vi "メイン.vi"() -> (2 "測定周期/ms":dbl, 3 "値転記用配列":T2[](array[typedef]))   [LabVIEW 2021] (continued)
                frame 8 {
                  n4757 = local write "測定新値\nリセット用 9"(w7303) -> ()
                  n4758 = local write "測定旧値 9"(w7303) -> ()
                }
                frame 9 {
                  n4759 = local write "測定新値\nリセット用 10"(w7304) -> ()
                  n4760 = local write "測定旧値 10"(w7304) -> ()
                }
                frame 10 {
                  n4761 = local write "測定新値\nリセット用 11"(w7305) -> ()
                  n4762 = local write "測定旧値 11"(w7305) -> ()
                }
                frame 11 {
                  n4763 = local write "測定新値\nリセット用 12"(w7306) -> ()
                  n4764 = local write "測定旧値 12"(w7306) -> ()
                }
              }
            }
          }
          frame #2 {
            # "⑤キュー"
            # "④グローバル_測定キャンセルボタンを\n対象測定新値がFalseならTrueにする"
            n4765 = case shown="TRUE" w7309 {
              tunnel: [_ w7319] -> w7313
              tunnel: w7312 -> [_ w7318]
              tunnel: [_ w7317] -> w7311
              tunnel: w7310 -> [_ w7316]
              tunnel: [w7314 w7315] -> w7308
              tunnel: [w7314 w7315] -> w7307
              frame False {
                w7314 = TRUE
              }
              frame True {
                w7315 = TRUE
                n4766 = Enqueue Element(queue=w7318, element="測定1", error in (no error)=w7316) -> (queue out=w7319:refnum<queue>, error out=w7317:errorcluster)  [unwired: 1 in, 1 out]
              }
            }
            n4767 = local write "G_メイン測定キャンセルボタン"(w7308) -> ()
            n4768 = global write "測定キャンセルボタン.vi" "グローバル_測定キャンセルボタン"(w7307) -> ()
          }
        }
        n4769 = for {
          N: 12 -> [_]
          tunnel: w7211 -> [w7225]
          i -> [w7226]
          n4770 = case shown="0, デフォルト" w7226 {
            tunnel: w7225 -> [w7227 w7228 w7229 w7230 w7231 w7232 w7233 w7234 w7235 w7236 w7237 w7238]
            frame 0, Default {
              n4771 = property on="メイン測定ボタン_単発 1" class="Bool (指定)"("DisabledEnum"=w7227) -> ()  [unwired: 2 in, 2 out]
              n4772 = property on="メイン測定ボタン_連続 1" class="Bool (指定)"("DisabledEnum"=w7227) -> ()  [unwired: 2 in, 2 out]
            }
            frame 1 {
              n4773 = property on="メイン測定ボタン_単発 2" class="Bool (指定)"("DisabledEnum"=w7228) -> ()  [unwired: 2 in, 2 out]
              n4774 = property on="メイン測定ボタン_連続 2" class="Bool (指定)"("DisabledEnum"=w7228) -> ()  [unwired: 2 in, 2 out]
            }
            frame 2 {
              n4775 = property on="メイン測定ボタン_単発 3" class="Bool (指定)"("DisabledEnum"=w7229) -> ()  [unwired: 2 in, 2 out]
              n4776 = property on="メイン測定ボタン_連続 3" class="Bool (指定)"("DisabledEnum"=w7229) -> ()  [unwired: 2 in, 2 out]
            }
            frame 3 {
              n4777 = property on="メイン測定ボタン_単発 4" class="Bool (指定)"("DisabledEnum"=w7230) -> ()  [unwired: 2 in, 2 out]
              n4778 = property on="メイン測定ボタン_連続 4" class="Bool (指定)"("DisabledEnum"=w7230) -> ()  [unwired: 2 in, 2 out]
            }
            frame 4 {
              n4779 = property on="メイン測定ボタン_単発 5" class="Bool (指定)"("DisabledEnum"=w7231) -> ()  [unwired: 2 in, 2 out]
              n4780 = property on="メイン測定ボタン_連続 5" class="Bool (指定)"("DisabledEnum"=w7231) -> ()  [unwired: 2 in, 2 out]
            }
            frame 5 {
              n4781 = property on="メイン測定ボタン_連続 6" class="Bool (指定)"("DisabledEnum"=w7232) -> ()  [unwired: 2 in, 2 out]
              n4782 = property on="メイン測定ボタン_単発 6" class="Bool (指定)"("DisabledEnum"=w7232) -> ()  [unwired: 2 in, 2 out]
            }
            frame 6 {
              n4783 = property on="メイン測定ボタン_連続 7" class="Bool (指定)"("DisabledEnum"=w7233) -> ()  [unwired: 2 in, 2 out]
              n4784 = property on="メイン測定ボタン_単発 7" class="Bool (指定)"("DisabledEnum"=w7233) -> ()  [unwired: 2 in, 2 out]
            }
            frame 7 {
              n4785 = property on="メイン測定ボタン_単発 8" class="Bool (指定)"("DisabledEnum"=w7234) -> ()  [unwired: 2 in, 2 out]
              n4786 = property on="メイン測定ボタン_連続 8" class="Bool (指定)"("DisabledEnum"=w7234) -> ()  [unwired: 2 in, 2 out]
            }
            frame 8 {
              n4787 = property on="メイン測定ボタン_単発 9" class="Bool (指定)"("DisabledEnum"=w7235) -> ()  [unwired: 2 in, 2 out]
              n4788 = property on="メイン測定ボタン_連続 9" class="Bool (指定)"("DisabledEnum"=w7235) -> ()  [unwired: 2 in, 2 out]
            }
            frame 9 {
              n4789 = property on="メイン測定ボタン_単発 10" class="Bool (指定)"("DisabledEnum"=w7236) -> ()  [unwired: 2 in, 2 out]
              n4790 = property on="メイン測定ボタン_連続 10" class="Bool (指定)"("DisabledEnum"=w7236) -> ()  [unwired: 2 in, 2 out]
            }
            frame 10 {
              n4791 = property on="メイン測定ボタン_単発 11" class="Bool (指定)"("DisabledEnum"=w7237) -> ()  [unwired: 2 in, 2 out]
              n4792 = property on="メイン測定ボタン_連続 11" class="Bool (指定)"("DisabledEnum"=w7237) -> ()  [unwired: 2 in, 2 out]
            }
            frame 11 {
              n4793 = property on="メイン測定ボタン_連続 12" class="Bool (指定)"("DisabledEnum"=w7238) -> ()  [unwired: 2 in, 2 out]
              n4794 = property on="メイン測定ボタン_単発 12" class="Bool (指定)"("DisabledEnum"=w7238) -> ()  [unwired: 2 in, 2 out]
            }
          }
        }
        n4795 = property on="TOPページへ" class="Bool"("DisabledEnum"=w7211) -> ()  [unwired: 2 in, 2 out]
        n4796 = property on="保存して終了" class="Bool"("DisabledEnum"=w7211) -> ()  [unwired: 2 in, 2 out]
        n4797 = property on="保存せずに" class="Bool"("DisabledEnum"=w7211) -> ()  [unwired: 2 in, 2 out]
      }
      event Value Change {
        w7322 = T8."Disabled" ("無効")
        # "※複製時\n①このボタンで操作する以外の\n測定旧値\n測定新値\nを複製して作る\n②ある分だけの\nを複製して作る\n③複製した番号未満のケースに\n②をコピーして置き換える\n(編集より楽な為)\n④はそのまま\n⑤測定新値の\nボタンが複製されているか確認\n⑥Ⅰ.初期設定の\n測定新値_リセットの初期化\nを必ず作る事\n⑦キュー"
        # "⑤"
        n4798 = event-data() -> ("NewVal"=w7331:T7)  [unwired: 1 in, 2 out]
        "測定新値 2" <- w7331
        n4799 = local read "書込周期/ms"() -> (w7321:dbl)
        n4800 = Wait (ms)(milliseconds to wait=w7321) -> ()  [unwired: 1 out]
        n4801 = flat-sequence {
          tunnel: [w7353] -> w7327
          tunnel: [w7352] -> w7326
          tunnel: [w7351] -> w7325
          tunnel: [w7350] -> w7324
          tunnel: w7331 -> [w7351]
          tunnel: w7332 -> [w7352]
          tunnel: w7334 -> [w7353]
          tunnel: [w7403] -> w7330
          tunnel: [w7402] -> w7329
          tunnel: [w7401] -> w7328
          tunnel: w7327 -> [w7403]
          tunnel: w7326 -> [w7402]
          tunnel: w7325 -> [w7401]
          tunnel: w7324 -> [w7399]
          tunnel: [w7424] -> w7335
          tunnel: [w7422] -> w7333
          tunnel: w7330 -> [w7423]
          tunnel: w7329 -> [w7421]
          tunnel: w7328 -> [w7420]
          frame #0 {
            w7350 = 32
            # "測定旧値・新値～32までTrueだったらMAX/MINグローバルリセット"
            # "①"
            n4802 = for {
              N: w7350 -> [_]
              i -> [w7354]
              n4803 = case shown="11" w7354 {
                frame 0, Default {
                  n4804 = local read "測定新値\nリセット用 1"() -> (w7355:bool)
                  n4805 = local read "測定旧値 1"() -> (w7356:bool)
                  n4806 = case shown="FALSE" w7355 {
                    frame False {
                    }
                    frame True {
                      n4807 = property on="MAX/MINグローバルリセット用" class="Arr (指定)"() -> ("Value"=w7357:string[][])  [unwired: 2 in, 2 out]
                      n4808 = global write "測定値MAXMIN_G.vi" "測定値MAX/MINグローバル"(w7357) -> ()
                    }
                  }
                  n4809 = case shown="FALSE" w7356 {
                    frame False {
                    }
                    frame True {
                      n4810 = property on="MAX/MINグローバルリセット用" class="Arr (指定)"() -> ("Value"=w7358:string[][])  [unwired: 2 in, 2 out]
                      n4811 = global write "測定値MAXMIN_G.vi" "測定値MAX/MINグローバル"(w7358) -> ()
                    }
                  }
                }
                frame 2 {
                  n4812 = local read "測定新値\nリセット用 3"() -> (w7359:bool)
                  n4813 = local read "測定旧値 3"() -> (w7360:bool)
                  n4814 = case shown="FALSE" w7359 {
                    frame False {
                    }
                    frame True {
                      n4815 = property on="MAX/MINグローバルリセット用" class="Arr (指定)"() -> ("Value"=w7361:string[][])  [unwired: 2 in, 2 out]
                      n4816 = global write "測定値MAXMIN_G.vi" "測定値MAX/MINグローバル"(w7361) -> ()
                    }
                  }
                  n4817 = case shown="FALSE" w7360 {
                    frame False {
                    }
                    frame True {
                      n4818 = property on="MAX/MINグローバルリセット用" class="Arr (指定)"() -> ("Value"=w7362:string[][])  [unwired: 2 in, 2 out]
                      n4819 = global write "測定値MAXMIN_G.vi" "測定値MAX/MINグローバル"(w7362) -> ()
                    }
                  }
                }
                frame 3 {
                  n4820 = local read "測定新値\nリセット用 4"() -> (w7363:bool)
                  n4821 = local read "測定旧値 4"() -> (w7364:bool)
                  n4822 = case shown="FALSE" w7363 {
                    frame False {
                    }
                    frame True {
                      n4823 = property on="MAX/MINグローバルリセット用" class="Arr (指定)"() -> ("Value"=w7365:string[][])  [unwired: 2 in, 2 out]
                      n4824 = global write "測定値MAXMIN_G.vi" "測定値MAX/MINグローバル"(w7365) -> ()
                    }
                  }
                  n4825 = case shown="FALSE" w7364 {
                    frame False {
                    }
                    frame True {
                      n4826 = property on="MAX/MINグローバルリセット用" class="Arr (指定)"() -> ("Value"=w7366:string[][])  [unwired: 2 in, 2 out]
                      n4827 = global write "測定値MAXMIN_G.vi" "測定値MAX/MINグローバル"(w7366) -> ()
                    }
                  }
                }
                frame 4 {
                  n4828 = local read "測定新値\nリセット用 5"() -> (w7367:bool)
                  n4829 = local read "測定旧値 5"() -> (w7368:bool)
                  n4830 = case shown="FALSE" w7367 {
                    frame False {
                    }
                    frame True {
                      n4831 = property on="MAX/MINグローバルリセット用" class="Arr (指定)"() -> ("Value"=w7369:string[][])  [unwired: 2 in, 2 out]
                      n4832 = global write "測定値MAXMIN_G.vi" "測定値MAX/MINグローバル"(w7369) -> ()
                    }
                  }
                  n4833 = case shown="FALSE" w7368 {
                    frame False {
                    }
                    frame True {
                      n4834 = property on="MAX/MINグローバルリセット用" class="Arr (指定)"() -> ("Value"=w7370:string[][])  [unwired: 2 in, 2 out]
                      n4835 = global write "測定値MAXMIN_G.vi" "測定値MAX/MINグローバル"(w7370) -> ()
                    }
                  }
                }
                frame 5 {
                  n4836 = local read "測定新値\nリセット用 6"() -> (w7371:bool)
                  n4837 = local read "測定旧値 6"() -> (w7372:bool)
                  n4838 = case shown="FALSE" w7371 {
                    frame False {
                    }
                    frame True {
                      n4839 = property on="MAX/MINグローバルリセット用" class="Arr (指定)"() -> ("Value"=w7373:string[][])  [unwired: 2 in, 2 out]
                      n4840 = global write "測定値MAXMIN_G.vi" "測定値MAX/MINグローバル"(w7373) -> ()
                    }
                  }
                  n4841 = case shown="FALSE" w7372 {
                    frame False {
                    }
                    frame True {
                      n4842 = property on="MAX/MINグローバルリセット用" class="Arr (指定)"() -> ("Value"=w7374:string[][])  [unwired: 2 in, 2 out]
                      n4843 = global write "測定値MAXMIN_G.vi" "測定値MAX/MINグローバル"(w7374) -> ()
                    }
                  }
                }
                frame 6 {
                  n4844 = local read "測定新値\nリセット用 7"() -> (w7375:bool)
                  n4845 = local read "測定旧値 7"() -> (w7376:bool)
                  n4846 = case shown="FALSE" w7375 {
                    frame False {
                    }
                    frame True {
                      n4847 = property on="MAX/MINグローバルリセット用" class="Arr (指定)"() -> ("Value"=w7377:string[][])  [unwired: 2 in, 2 out]
                      n4848 = global write "測定値MAXMIN_G.vi" "測定値MAX/MINグローバル"(w7377) -> ()
                    }
                  }
                  n4849 = case shown="FALSE" w7376 {
                    frame False {
                    }
                    frame True {
                      n4850 = property on="MAX/MINグローバルリセット用" class="Arr (指定)"() -> ("Value"=w7378:string[][])  [unwired: 2 in, 2 out]
                      n4851 = global write "測定値MAXMIN_G.vi" "測定値MAX/MINグローバル"(w7378) -> ()
                    }
                  }
                }
                frame 7 {
                  n4852 = local read "測定新値\nリセット用 8"() -> (w7379:bool)
                  n4853 = local read "測定旧値 8"() -> (w7380:bool)
                  n4854 = case shown="FALSE" w7379 {
                    frame False {
                    }
                    frame True {
                      n4855 = property on="MAX/MINグローバルリセット用" class="Arr (指定)"() -> ("Value"=w7381:string[][])  [unwired: 2 in, 2 out]
                      n4856 = global write "測定値MAXMIN_G.vi" "測定値MAX/MINグローバル"(w7381) -> ()
                    }
                  }
                  n4857 = case shown="FALSE" w7380 {
                    frame False {
                    }
                    frame True {
                      n4858 = property on="MAX/MINグローバルリセット用" class="Arr (指定)"() -> ("Value"=w7382:string[][])  [unwired: 2 in, 2 out]
                      n4859 = global write "測定値MAXMIN_G.vi" "測定値MAX/MINグローバル"(w7382) -> ()
                    }
                  }
                }
                frame 8 {
                  n4860 = local read "測定新値\nリセット用 9"() -> (w7383:bool)
                  n4861 = local read "測定旧値 9"() -> (w7384:bool)
                  n4862 = case shown="TRUE" w7383 {
                    frame False {
                    }
                    frame True {
                      n4863 = property on="MAX/MINグローバルリセット用" class="Arr (指定)"() -> ("Value"=w7385:string[][])  [unwired: 2 in, 2 out]
                      n4864 = global write "測定値MAXMIN_G.vi" "測定値MAX/MINグローバル"(w7385) -> ()
                    }
                  }
                  n4865 = case shown="TRUE" w7384 {
                    frame False {
                    }
                    frame True {
                      n4866 = property on="MAX/MINグローバルリセット用" class="Arr (指定)"() -> ("Value"=w7386:string[][])  [unwired: 2 in, 2 out]
                      n4867 = global write "測定値MAXMIN_G.vi" "測定値MAX/MINグローバル"(w7386) -> ()
                    }
                  }
                }
                frame 9 {
                  n4868 = local read "測定新値\nリセット用 10"() -> (w7387:bool)
                  n4869 = local read "測定旧値 10"() -> (w7388:bool)
                  n4870 = case shown="TRUE" w7387 {
                    frame False {
                    }
                    frame True {
                      n4871 = property on="MAX/MINグローバルリセット用" class="Arr (指定)"() -> ("Value"=w7389:string[][])  [unwired: 2 in, 2 out]
                      n4872 = global write "測定値MAXMIN_G.vi" "測定値MAX/MINグローバル"(w7389) -> ()
                    }
                  }
                  n4873 = case shown="TRUE" w7388 {
                    frame False {
                    }
                    frame True {
                      n4874 = property on="MAX/MINグローバルリセット用" class="Arr (指定)"() -> ("Value"=w7390:string[][])  [unwired: 2 in, 2 out]
                      n4875 = global write "測定値MAXMIN_G.vi" "測定値MAX/MINグローバル"(w7390) -> ()
                    }
                  }
                }
                frame 10 {
                  n4876 = local read "測定新値\nリセット用 11"() -> (w7391:bool)
                  n4877 = local read "測定旧値 11"() -> (w7392:bool)
                  n4878 = case shown="TRUE" w7391 {
                    frame False {
                    }
                    frame True {
                      n4879 = property on="MAX/MINグローバルリセット用" class="Arr (指定)"() -> ("Value"=w7393:string[][])  [unwired: 2 in, 2 out]
                      n4880 = global write "測定値MAXMIN_G.vi" "測定値MAX/MINグローバル"(w7393) -> ()
                    }
                  }
                  n4881 = case shown="TRUE" w7392 {
                    frame False {
                    }
                    frame True {
                      n4882 = property on="MAX/MINグローバルリセット用" class="Arr (指定)"() -> ("Value"=w7394:string[][])  [unwired: 2 in, 2 out]
                      n4883 = global write "測定値MAXMIN_G.vi" "測定値MAX/MINグローバル"(w7394) -> ()
                    }
                  }
                }
                frame 11 {
                  n4884 = local read "測定新値\nリセット用 12"() -> (w7395:bool)
                  n4885 = local read "測定旧値 12"() -> (w7396:bool)
                  n4886 = case shown="TRUE" w7395 {
                    frame False {
                    }
                    frame True {
                      n4887 = property on="MAX/MINグローバルリセット用" class="Arr (指定)"() -> ("Value"=w7397:string[][])  [unwired: 2 in, 2 out]
                      n4888 = global write "測定値MAXMIN_G.vi" "測定値MAX/MINグローバル"(w7397) -> ()
                    }
                  }
                  n4889 = case shown="TRUE" w7396 {
                    frame False {
                    }
                    frame True {
                      n4890 = property on="MAX/MINグローバルリセット用" class="Arr (指定)"() -> ("Value"=w7398:string[][])  [unwired: 2 in, 2 out]
                      n4891 = global write "測定値MAXMIN_G.vi" "測定値MAX/MINグローバル"(w7398) -> ()
                    }
                  }
                }
                frame 1 {
                }
              }
            }
          }
          frame #1 {
            w7400 = FALSE
            # "②測定新規リセット用、測定旧値のリセット"
            n4892 = for {
              N: w7399 -> [_]
              tunnel: w7400 -> [w7404]
              i -> [w7405]
              n4893 = case shown="11" w7405 {
                tunnel: w7404 -> [w7406 w7407 w7408 w7409 w7410 w7411 w7412 w7413 w7414 w7415 w7416 w7417]
                frame 0, Default {
                  n4894 = local write "測定新値\nリセット用 1"(w7406) -> ()
                  n4895 = local write "測定旧値 1"(w7406) -> ()
                }
                frame 1 {
                  n4896 = local write "測定新値\nリセット用 2"(w7407) -> ()
                  n4897 = local write "測定旧値 2"(w7407) -> ()
                }
                frame 2 {
                  n4898 = local write "測定新値\nリセット用 3"(w7408) -> ()
                  n4899 = local write "測定旧値 3"(w7408) -> ()
                }
                frame 3 {
                  n4900 = local write "測定新値\nリセット用 4"(w7409) -> ()
                  n4901 = local write "測定旧値 4"(w7409) -> ()
                }
                frame 4 {
                  n4902 = local write "測定新値\nリセット用 5"(w7410) -> ()
                  n4903 = local write "測定旧値 5"(w7410) -> ()
                }
                frame 5 {
                  n4904 = local write "測定新値\nリセット用 6"(w7411) -> ()
                  n4905 = local write "測定旧値 6"(w7411) -> ()
                }
                frame 6 {
                  n4906 = local write "測定新値\nリセット用 7"(w7412) -> ()
                  n4907 = local write "測定旧値 7"(w7412) -> ()
                }
                frame 7 {
                  n4908 = local write "測定新値\nリセット用 8"(w7413) -> ()
                  n4909 = local write "測定旧値 8"(w7413) -> ()
                }
                frame 8 {
                  n4910 = local write "測定新値\nリセット用 9"(w7414) -> ()
                  n4911 = local write "測定旧値 9"(w7414) -> ()
                }
                frame 9 {
                  n4912 = local write "測定新値\nリセット用 10"(w7415) -> ()
                  n4913 = local write "測定旧値 10"(w7415) -> ()
                }
                frame 10 {
                  n4914 = local write "測定新値\nリセット用 11"(w7416) -> ()
                  n4915 = local write "測定旧値 11"(w7416) -> ()
                }
                frame 11 {
                  n4916 = local write "測定新値\nリセット用 12"(w7417) -> ()
                  n4917 = local write "測定旧値 12"(w7417) -> ()
                }
              }
            }
            n4918 = global write "測定キャンセルボタン.vi" "グローバル_測定キャンセルボタン"(w7400) -> ()
            n4919 = local write "G_メイン測定キャンセルボタン"(w7400) -> ()
          }
          frame #2 {
            # "⑦キュー"
            # "④グローバル_測定キャンセルボタンを\n対象測定新値がFalseならTrueにする"
            n4920 = case shown="TRUE" w7420 {
              tunnel: [_ w7430] -> w7424
              tunnel: w7423 -> [_ w7429]
              tunnel: [_ w7428] -> w7422
              tunnel: w7421 -> [_ w7427]
              tunnel: [w7425 w7426] -> w7419
              tunnel: [w7425 w7426] -> w7418
              frame False {
                w7425 = TRUE
              }
              frame True {
                w7426 = TRUE
                n4921 = Enqueue Element(queue=w7429, element="測定2", error in (no error)=w7427) -> (queue out=w7430:refnum<queue>, error out=w7428:errorcluster)  [unwired: 1 in, 1 out]
              }
            }
            n4922 = local write "G_メイン測定キャンセルボタン"(w7419) -> ()
            n4923 = global write "測定キャンセルボタン.vi" "グローバル_測定キャンセルボタン"(w7418) -> ()
          }
        }
        n4924 = for {
          N: 12 -> [_]
          tunnel: w7322 -> [w7336]
          i -> [w7337]
          n4925 = case shown="11" w7337 {
            tunnel: w7336 -> [w7338 w7339 w7340 w7341 w7342 w7343 w7344 w7345 w7346 w7347 w7348 w7349]
            frame 0, Default {
              n4926 = property on="メイン測定ボタン_単発 1" class="Bool (指定)"("DisabledEnum"=w7338) -> ()  [unwired: 2 in, 2 out]
              n4927 = property on="メイン測定ボタン_連続 1" class="Bool (指定)"("DisabledEnum"=w7338) -> ()  [unwired: 2 in, 2 out]
            }
            frame 1 {
              n4928 = property on="メイン測定ボタン_単発 2" class="Bool (指定)"("DisabledEnum"=w7339) -> ()  [unwired: 2 in, 2 out]
              n4929 = property on="メイン測定ボタン_連続 2" class="Bool (指定)"("DisabledEnum"=w7339) -> ()  [unwired: 2 in, 2 out]
            }
            frame 2 {
              n4930 = property on="メイン測定ボタン_単発 3" class="Bool (指定)"("DisabledEnum"=w7340) -> ()  [unwired: 2 in, 2 out]
              n4931 = property on="メイン測定ボタン_連続 3" class="Bool (指定)"("DisabledEnum"=w7340) -> ()  [unwired: 2 in, 2 out]
            }
            frame 3 {
              n4932 = property on="メイン測定ボタン_単発 4" class="Bool (指定)"("DisabledEnum"=w7341) -> ()  [unwired: 2 in, 2 out]
              n4933 = property on="メイン測定ボタン_連続 4" class="Bool (指定)"("DisabledEnum"=w7341) -> ()  [unwired: 2 in, 2 out]
            }
            frame 4 {
              n4934 = property on="メイン測定ボタン_単発 5" class="Bool (指定)"("DisabledEnum"=w7342) -> ()  [unwired: 2 in, 2 out]
              n4935 = property on="メイン測定ボタン_連続 5" class="Bool (指定)"("DisabledEnum"=w7342) -> ()  [unwired: 2 in, 2 out]
            }
            frame 5 {
              n4936 = property on="メイン測定ボタン_連続 6" class="Bool (指定)"("DisabledEnum"=w7343) -> ()  [unwired: 2 in, 2 out]
              n4937 = property on="メイン測定ボタン_単発 6" class="Bool (指定)"("DisabledEnum"=w7343) -> ()  [unwired: 2 in, 2 out]
            }
            frame 6 {
              n4938 = property on="メイン測定ボタン_連続 7" class="Bool (指定)"("DisabledEnum"=w7344) -> ()  [unwired: 2 in, 2 out]
              n4939 = property on="メイン測定ボタン_単発 7" class="Bool (指定)"("DisabledEnum"=w7344) -> ()  [unwired: 2 in, 2 out]
            }
            frame 7 {
              n4940 = property on="メイン測定ボタン_単発 8" class="Bool (指定)"("DisabledEnum"=w7345) -> ()  [unwired: 2 in, 2 out]
              n4941 = property on="メイン測定ボタン_連続 8" class="Bool (指定)"("DisabledEnum"=w7345) -> ()  [unwired: 2 in, 2 out]
            }
            frame 8 {
              n4942 = property on="メイン測定ボタン_単発 9" class="Bool (指定)"("DisabledEnum"=w7346) -> ()  [unwired: 2 in, 2 out]
              n4943 = property on="メイン測定ボタン_連続 9" class="Bool (指定)"("DisabledEnum"=w7346) -> ()  [unwired: 2 in, 2 out]
            }
            frame 9 {
              n4944 = property on="メイン測定ボタン_単発 10" class="Bool (指定)"("DisabledEnum"=w7347) -> ()  [unwired: 2 in, 2 out]
              n4945 = property on="メイン測定ボタン_連続 10" class="Bool (指定)"("DisabledEnum"=w7347) -> ()  [unwired: 2 in, 2 out]
            }
            frame 10 {
              n4946 = property on="メイン測定ボタン_単発 11" class="Bool (指定)"("DisabledEnum"=w7348) -> ()  [unwired: 2 in, 2 out]
              n4947 = property on="メイン測定ボタン_連続 11" class="Bool (指定)"("DisabledEnum"=w7348) -> ()  [unwired: 2 in, 2 out]
            }
            frame 11 {
              n4948 = property on="メイン測定ボタン_連続 12" class="Bool (指定)"("DisabledEnum"=w7349) -> ()  [unwired: 2 in, 2 out]
              n4949 = property on="メイン測定ボタン_単発 12" class="Bool (指定)"("DisabledEnum"=w7349) -> ()  [unwired: 2 in, 2 out]
            }
          }
        }
        n4950 = property on="TOPページへ" class="Bool"("DisabledEnum"=w7322) -> ()  [unwired: 2 in, 2 out]
        n4951 = property on="保存して終了" class="Bool"("DisabledEnum"=w7322) -> ()  [unwired: 2 in, 2 out]
        n4952 = property on="保存せずに" class="Bool"("DisabledEnum"=w7322) -> ()  [unwired: 2 in, 2 out]
      }
      event Value Change {
        w7433 = T8."Disabled" ("無効")
        # "⑤"
        # "※複製時\n①このボタンで操作する以外の\n測定旧値\n測定新値\nを複製して作る\n②ある分だけの\n測定旧値\nを複製して作る\n③ある分だけの\n測定旧値\nを複製して作る\n④はそのまま\n⑤測定新値の\nボタンが複製されているか確認\n⑥Ⅰ.初期設定の\n測定新値_リセットの初期化\nを必ず作る事\n⑦キュー"
        n4953 = event-data() -> ("NewVal"=w7442:T7)  [unwired: 1 in, 2 out]
        "測定新値 3" <- w7442
        n4954 = local read "書込周期/ms"() -> (w7432:dbl)
        n4955 = Wait (ms)(milliseconds to wait=w7432) -> ()  [unwired: 1 out]
        n4956 = flat-sequence {
          tunnel: w7442 -> [w7462]
          tunnel: w7443 -> [w7463]
          tunnel: w7445 -> [w7464]
          tunnel: [w7464] -> w7438
          tunnel: [w7463] -> w7437
          tunnel: [w7462] -> w7436
          tunnel: [w7461] -> w7435
          tunnel: [w7514] -> w7441
          tunnel: [w7513] -> w7440
          tunnel: [w7512] -> w7439
          tunnel: w7435 -> [w7510]
          tunnel: w7436 -> [w7512]
          tunnel: w7437 -> [w7513]
          tunnel: w7438 -> [w7514]
          tunnel: [w7535] -> w7446
          tunnel: [w7533] -> w7444
          tunnel: w7441 -> [w7534]
          tunnel: w7440 -> [w7532]
          tunnel: w7439 -> [w7531]
          frame #0 {
            w7461 = 32
            # "測定旧値・新値～32までTrueだったらMAX/MINグローバルリセット"
            # "①"
            n4957 = for {
              N: w7461 -> [_]
              i -> [w7465]
              n4958 = case shown="11" w7465 {
                frame 0, Default {
                  n4959 = local read "測定新値\nリセット用 1"() -> (w7466:bool)
                  n4960 = local read "測定旧値 1"() -> (w7467:bool)
                  n4961 = case shown="TRUE" w7466 {
                    frame False {
                    }
                    frame True {
                      n4962 = property on="MAX/MINグローバルリセット用" class="Arr (指定)"() -> ("Value"=w7468:string[][])  [unwired: 2 in, 2 out]
                      n4963 = global write "測定値MAXMIN_G.vi" "測定値MAX/MINグローバル"(w7468) -> ()
                    }
                  }
                  n4964 = case shown="TRUE" w7467 {
                    frame False {
                    }
                    frame True {
                      n4965 = property on="MAX/MINグローバルリセット用" class="Arr (指定)"() -> ("Value"=w7469:string[][])  [unwired: 2 in, 2 out]
                      n4966 = global write "測定値MAXMIN_G.vi" "測定値MAX/MINグローバル"(w7469) -> ()
                    }
                  }
                }
                frame 1 {
                  n4967 = local read "測定新値\nリセット用 2"() -> (w7470:bool)
                  n4968 = local read "測定旧値 2"() -> (w7471:bool)
                  n4969 = case shown="TRUE" w7470 {
                    frame False {
                    }
                    frame True {
                      n4970 = property on="MAX/MINグローバルリセット用" class="Arr (指定)"() -> ("Value"=w7472:string[][])  [unwired: 2 in, 2 out]
                      n4971 = global write "測定値MAXMIN_G.vi" "測定値MAX/MINグローバル"(w7472) -> ()
                    }
                  }
                  n4972 = case shown="TRUE" w7471 {
                    frame False {
                    }
                    frame True {
                      n4973 = property on="MAX/MINグローバルリセット用" class="Arr (指定)"() -> ("Value"=w7473:string[][])  [unwired: 2 in, 2 out]
                      n4974 = global write "測定値MAXMIN_G.vi" "測定値MAX/MINグローバル"(w7473) -> ()
                    }
                  }
                }
                frame 3 {
                  n4975 = local read "測定新値\nリセット用 4"() -> (w7474:bool)
                  n4976 = local read "測定旧値 4"() -> (w7475:bool)
                  n4977 = case shown="TRUE" w7474 {
                    frame False {
                    }
                    frame True {
                      n4978 = property on="MAX/MINグローバルリセット用" class="Arr (指定)"() -> ("Value"=w7476:string[][])  [unwired: 2 in, 2 out]
                      n4979 = global write "測定値MAXMIN_G.vi" "測定値MAX/MINグローバル"(w7476) -> ()
                    }
                  }
                  n4980 = case shown="TRUE" w7475 {
                    frame False {
                    }
                    frame True {
                      n4981 = property on="MAX/MINグローバルリセット用" class="Arr (指定)"() -> ("Value"=w7477:string[][])  [unwired: 2 in, 2 out]
                      n4982 = global write "測定値MAXMIN_G.vi" "測定値MAX/MINグローバル"(w7477) -> ()
                    }
                  }
                }
                frame 4 {
                  n4983 = local read "測定新値\nリセット用 5"() -> (w7478:bool)
                  n4984 = local read "測定旧値 5"() -> (w7479:bool)
                  n4985 = case shown="TRUE" w7478 {
                    frame False {
                    }
                    frame True {
                      n4986 = property on="MAX/MINグローバルリセット用" class="Arr (指定)"() -> ("Value"=w7480:string[][])  [unwired: 2 in, 2 out]
                      n4987 = global write "測定値MAXMIN_G.vi" "測定値MAX/MINグローバル"(w7480) -> ()
                    }
                  }
                  n4988 = case shown="TRUE" w7479 {
                    frame False {
                    }
                    frame True {
                      n4989 = property on="MAX/MINグローバルリセット用" class="Arr (指定)"() -> ("Value"=w7481:string[][])  [unwired: 2 in, 2 out]
                      n4990 = global write "測定値MAXMIN_G.vi" "測定値MAX/MINグローバル"(w7481) -> ()
                    }
                  }
                }
                frame 5 {
                  n4991 = local read "測定新値\nリセット用 6"() -> (w7482:bool)
                  n4992 = local read "測定旧値 6"() -> (w7483:bool)
                  n4993 = case shown="TRUE" w7482 {
                    frame False {
                    }
                    frame True {
                      n4994 = property on="MAX/MINグローバルリセット用" class="Arr (指定)"() -> ("Value"=w7484:string[][])  [unwired: 2 in, 2 out]
                      n4995 = global write "測定値MAXMIN_G.vi" "測定値MAX/MINグローバル"(w7484) -> ()
                    }
                  }
                  n4996 = case shown="TRUE" w7483 {
                    frame False {
                    }
                    frame True {
                      n4997 = property on="MAX/MINグローバルリセット用" class="Arr (指定)"() -> ("Value"=w7485:string[][])  [unwired: 2 in, 2 out]
                      n4998 = global write "測定値MAXMIN_G.vi" "測定値MAX/MINグローバル"(w7485) -> ()
                    }
                  }
                }
                frame 6 {
                  n4999 = local read "測定新値\nリセット用 7"() -> (w7486:bool)
                  n5000 = local read "測定旧値 7"() -> (w7487:bool)
                  n5001 = case shown="TRUE" w7486 {
                    frame False {
                    }
                    frame True {
                      n5002 = property on="MAX/MINグローバルリセット用" class="Arr (指定)"() -> ("Value"=w7488:string[][])  [unwired: 2 in, 2 out]
                      n5003 = global write "測定値MAXMIN_G.vi" "測定値MAX/MINグローバル"(w7488) -> ()
                    }
                  }
                  n5004 = case shown="TRUE" w7487 {
                    frame False {
                    }
                    frame True {
                      n5005 = property on="MAX/MINグローバルリセット用" class="Arr (指定)"() -> ("Value"=w7489:string[][])  [unwired: 2 in, 2 out]
                      n5006 = global write "測定値MAXMIN_G.vi" "測定値MAX/MINグローバル"(w7489) -> ()
                    }
                  }
                }
                frame 7 {
                  n5007 = local read "測定新値\nリセット用 8"() -> (w7490:bool)
                  n5008 = local read "測定旧値 8"() -> (w7491:bool)
                  n5009 = case shown="TRUE" w7490 {
                    frame False {
                    }
                    frame True {
                      n5010 = property on="MAX/MINグローバルリセット用" class="Arr (指定)"() -> ("Value"=w7492:string[][])  [unwired: 2 in, 2 out]
                      n5011 = global write "測定値MAXMIN_G.vi" "測定値MAX/MINグローバル"(w7492) -> ()
                    }
                  }
                  n5012 = case shown="TRUE" w7491 {
                    frame False {
                    }
                    frame True {
                      n5013 = property on="MAX/MINグローバルリセット用" class="Arr (指定)"() -> ("Value"=w7493:string[][])  [unwired: 2 in, 2 out]
                      n5014 = global write "測定値MAXMIN_G.vi" "測定値MAX/MINグローバル"(w7493) -> ()
                    }
                  }
                }
                frame 8 {
                  n5015 = local read "測定新値\nリセット用 9"() -> (w7494:bool)
                  n5016 = local read "測定旧値 9"() -> (w7495:bool)
                  n5017 = case shown="TRUE" w7494 {
                    frame False {
                    }
                    frame True {
                      n5018 = property on="MAX/MINグローバルリセット用" class="Arr (指定)"() -> ("Value"=w7496:string[][])  [unwired: 2 in, 2 out]
                      n5019 = global write "測定値MAXMIN_G.vi" "測定値MAX/MINグローバル"(w7496) -> ()
                    }
                  }
                  n5020 = case shown="TRUE" w7495 {
                    frame False {
                    }
                    frame True {
                      n5021 = property on="MAX/MINグローバルリセット用" class="Arr (指定)"() -> ("Value"=w7497:string[][])  [unwired: 2 in, 2 out]
                      n5022 = global write "測定値MAXMIN_G.vi" "測定値MAX/MINグローバル"(w7497) -> ()
                    }
                  }
                }
                frame 9 {
                  n5023 = local read "測定新値\nリセット用 10"() -> (w7498:bool)
                  n5024 = local read "測定旧値 10"() -> (w7499:bool)
                  n5025 = case shown="TRUE" w7498 {
                    frame False {
                    }
                    frame True {
                      n5026 = property on="MAX/MINグローバルリセット用" class="Arr (指定)"() -> ("Value"=w7500:string[][])  [unwired: 2 in, 2 out]
                      n5027 = global write "測定値MAXMIN_G.vi" "測定値MAX/MINグローバル"(w7500) -> ()
                    }
                  }
                  n5028 = case shown="TRUE" w7499 {
                    frame False {
                    }
                    frame True {
                      n5029 = property on="MAX/MINグローバルリセット用" class="Arr (指定)"() -> ("Value"=w7501:string[][])  [unwired: 2 in, 2 out]
                      n5030 = global write "測定値MAXMIN_G.vi" "測定値MAX/MINグローバル"(w7501) -> ()
                    }
                  }
                }
                frame 10 {
                  n5031 = local read "測定新値\nリセット用 11"() -> (w7502:bool)
                  n5032 = local read "測定旧値 11"() -> (w7503:bool)
                  n5033 = case shown="TRUE" w7502 {
                    frame False {
                    }
                    frame True {
                      n5034 = property on="MAX/MINグローバルリセット用" class="Arr (指定)"() -> ("Value"=w7504:string[][])  [unwired: 2 in, 2 out]
                      n5035 = global write "測定値MAXMIN_G.vi" "測定値MAX/MINグローバル"(w7504) -> ()
                    }
                  }
                  n5036 = case shown="TRUE" w7503 {
                    frame False {
                    }
                    frame True {
                      n5037 = property on="MAX/MINグローバルリセット用" class="Arr (指定)"() -> ("Value"=w7505:string[][])  [unwired: 2 in, 2 out]
                      n5038 = global write "測定値MAXMIN_G.vi" "測定値MAX/MINグローバル"(w7505) -> ()
                    }
                  }
                }
                frame 11 {
                  n5039 = local read "測定新値\nリセット用 12"() -> (w7506:bool)
                  n5040 = local read "測定旧値 12"() -> (w7507:bool)
                  n5041 = case shown="TRUE" w7506 {
                    frame False {
                    }
                    frame True {
                      n5042 = property on="MAX/MINグローバルリセット用" class="Arr (指定)"() -> ("Value"=w7508:string[][])  [unwired: 2 in, 2 out]
                      n5043 = global write "測定値MAXMIN_G.vi" "測定値MAX/MINグローバル"(w7508) -> ()
                    }
                  }
                  n5044 = case shown="TRUE" w7507 {
                    frame False {
                    }
                    frame True {
                      n5045 = property on="MAX/MINグローバルリセット用" class="Arr (指定)"() -> ("Value"=w7509:string[][])  [unwired: 2 in, 2 out]
                      n5046 = global write "測定値MAXMIN_G.vi" "測定値MAX/MINグローバル"(w7509) -> ()
                    }
                  }
                }
              }
            }
          }
          frame #1 {
            w7511 = FALSE
            # "②測定新規リセット用、測定旧値のリセット"
            n5047 = global write "測定キャンセルボタン.vi" "グローバル_測定キャンセルボタン"(w7511) -> ()
            n5048 = local write "G_メイン測定キャンセルボタン"(w7511) -> ()
            n5049 = for {
              N: w7510 -> [_]
              tunnel: w7511 -> [w7515]
              i -> [w7516]
              n5050 = case shown="11" w7516 {
                tunnel: w7515 -> [w7517 w7518 w7519 w7520 w7521 w7522 w7523 w7524 w7525 w7526 w7527 w7528]
                frame 0, Default {
                  n5051 = local write "測定新値\nリセット用 1"(w7517) -> ()
                  n5052 = local write "測定旧値 1"(w7517) -> ()
                }
                frame 1 {
                  n5053 = local write "測定新値\nリセット用 2"(w7518) -> ()
                  n5054 = local write "測定旧値 2"(w7518) -> ()
                }
                frame 2 {
                  n5055 = local write "測定新値\nリセット用 3"(w7519) -> ()
                  n5056 = local write "測定旧値 3"(w7519) -> ()
                }
                frame 3 {
                  n5057 = local write "測定新値\nリセット用 4"(w7520) -> ()
                  n5058 = local write "測定旧値 4"(w7520) -> ()
                }
                frame 4 {
                  n5059 = local write "測定新値\nリセット用 5"(w7521) -> ()
                  n5060 = local write "測定旧値 5"(w7521) -> ()
                }
                frame 5 {
                  n5061 = local write "測定新値\nリセット用 6"(w7522) -> ()
                  n5062 = local write "測定旧値 6"(w7522) -> ()
                }
                frame 6 {
                  n5063 = local write "測定新値\nリセット用 7"(w7523) -> ()
                  n5064 = local write "測定旧値 7"(w7523) -> ()
                }
                frame 7 {
                  n5065 = local write "測定新値\nリセット用 8"(w7524) -> ()
                  n5066 = local write "測定旧値 8"(w7524) -> ()
                }
                frame 8 {
                  n5067 = local write "測定新値\nリセット用 9"(w7525) -> ()
                  n5068 = local write "測定旧値 9"(w7525) -> ()
                }
                frame 9 {
                  n5069 = local write "測定新値\nリセット用 10"(w7526) -> ()
                  n5070 = local write "測定旧値 10"(w7526) -> ()
                }
                frame 10 {
                  n5071 = local write "測定新値\nリセット用 11"(w7527) -> ()
                  n5072 = local write "測定旧値 11"(w7527) -> ()
                }
                frame 11 {
                  n5073 = local write "測定新値\nリセット用 12"(w7528) -> ()
                  n5074 = local write "測定旧値 12"(w7528) -> ()
                }
              }
            }
          }
          frame #2 {
            # "⑦キュー"
            # "④グローバル_測定キャンセルボタンを\n対象測定新値がFalseならTrueにする"
            n5075 = case shown="TRUE" w7531 {
              tunnel: [_ w7541] -> w7535
              tunnel: w7534 -> [_ w7540]
              tunnel: [_ w7539] -> w7533
              tunnel: w7532 -> [_ w7538]
              tunnel: [w7536 w7537] -> w7530
              tunnel: [w7536 w7537] -> w7529
              frame False {
                w7536 = TRUE
              }
              frame True {
                w7537 = TRUE
                n5076 = Enqueue Element(queue=w7540, element="測定3", error in (no error)=w7538) -> (queue out=w7541:refnum<queue>, error out=w7539:errorcluster)  [unwired: 1 in, 1 out]
              }
            }
            n5077 = local write "G_メイン測定キャンセルボタン"(w7530) -> ()
            n5078 = global write "測定キャンセルボタン.vi" "グローバル_測定キャンセルボタン"(w7529) -> ()
          }
        }
        n5079 = for {
          N: 12 -> [_]
          tunnel: w7433 -> [w7447]
          i -> [w7448]
          n5080 = case shown="11" w7448 {
            tunnel: w7447 -> [w7449 w7450 w7451 w7452 w7453 w7454 w7455 w7456 w7457 w7458 w7459 w7460]
            frame 0, Default {
              n5081 = property on="メイン測定ボタン_単発 1" class="Bool (指定)"("DisabledEnum"=w7449) -> ()  [unwired: 2 in, 2 out]
              n5082 = property on="メイン測定ボタン_連続 1" class="Bool (指定)"("DisabledEnum"=w7449) -> ()  [unwired: 2 in, 2 out]
            }
            frame 1 {
              n5083 = property on="メイン測定ボタン_単発 2" class="Bool (指定)"("DisabledEnum"=w7450) -> ()  [unwired: 2 in, 2 out]
              n5084 = property on="メイン測定ボタン_連続 2" class="Bool (指定)"("DisabledEnum"=w7450) -> ()  [unwired: 2 in, 2 out]
            }
            frame 2 {
              n5085 = property on="メイン測定ボタン_単発 3" class="Bool (指定)"("DisabledEnum"=w7451) -> ()  [unwired: 2 in, 2 out]
              n5086 = property on="メイン測定ボタン_連続 3" class="Bool (指定)"("DisabledEnum"=w7451) -> ()  [unwired: 2 in, 2 out]
            }
            frame 3 {
              n5087 = property on="メイン測定ボタン_単発 4" class="Bool (指定)"("DisabledEnum"=w7452) -> ()  [unwired: 2 in, 2 out]
              n5088 = property on="メイン測定ボタン_連続 4" class="Bool (指定)"("DisabledEnum"=w7452) -> ()  [unwired: 2 in, 2 out]
            }
            frame 4 {
              n5089 = property on="メイン測定ボタン_単発 5" class="Bool (指定)"("DisabledEnum"=w7453) -> ()  [unwired: 2 in, 2 out]
              n5090 = property on="メイン測定ボタン_連続 5" class="Bool (指定)"("DisabledEnum"=w7453) -> ()  [unwired: 2 in, 2 out]
            }
            frame 5 {
              n5091 = property on="メイン測定ボタン_連続 6" class="Bool (指定)"("DisabledEnum"=w7454) -> ()  [unwired: 2 in, 2 out]
              n5092 = property on="メイン測定ボタン_単発 6" class="Bool (指定)"("DisabledEnum"=w7454) -> ()  [unwired: 2 in, 2 out]
            }
            frame 6 {
              n5093 = property on="メイン測定ボタン_連続 7" class="Bool (指定)"("DisabledEnum"=w7455) -> ()  [unwired: 2 in, 2 out]
              n5094 = property on="メイン測定ボタン_単発 7" class="Bool (指定)"("DisabledEnum"=w7455) -> ()  [unwired: 2 in, 2 out]
            }
            frame 7 {
              n5095 = property on="メイン測定ボタン_単発 8" class="Bool (指定)"("DisabledEnum"=w7456) -> ()  [unwired: 2 in, 2 out]
              n5096 = property on="メイン測定ボタン_連続 8" class="Bool (指定)"("DisabledEnum"=w7456) -> ()  [unwired: 2 in, 2 out]
            }
            frame 8 {
              n5097 = property on="メイン測定ボタン_単発 9" class="Bool (指定)"("DisabledEnum"=w7457) -> ()  [unwired: 2 in, 2 out]
              n5098 = property on="メイン測定ボタン_連続 9" class="Bool (指定)"("DisabledEnum"=w7457) -> ()  [unwired: 2 in, 2 out]
            }
            frame 9 {
              n5099 = property on="メイン測定ボタン_単発 10" class="Bool (指定)"("DisabledEnum"=w7458) -> ()  [unwired: 2 in, 2 out]
              n5100 = property on="メイン測定ボタン_連続 10" class="Bool (指定)"("DisabledEnum"=w7458) -> ()  [unwired: 2 in, 2 out]
            }
            frame 10 {
              n5101 = property on="メイン測定ボタン_単発 11" class="Bool (指定)"("DisabledEnum"=w7459) -> ()  [unwired: 2 in, 2 out]
              n5102 = property on="メイン測定ボタン_連続 11" class="Bool (指定)"("DisabledEnum"=w7459) -> ()  [unwired: 2 in, 2 out]
            }
            frame 11 {
              n5103 = property on="メイン測定ボタン_連続 12" class="Bool (指定)"("DisabledEnum"=w7460) -> ()  [unwired: 2 in, 2 out]
              n5104 = property on="メイン測定ボタン_単発 12" class="Bool (指定)"("DisabledEnum"=w7460) -> ()  [unwired: 2 in, 2 out]
            }
          }
        }
        n5105 = property on="TOPページへ" class="Bool"("DisabledEnum"=w7433) -> ()  [unwired: 2 in, 2 out]
        n5106 = property on="保存して終了" class="Bool"("DisabledEnum"=w7433) -> ()  [unwired: 2 in, 2 out]
        n5107 = property on="保存せずに" class="Bool"("DisabledEnum"=w7433) -> ()  [unwired: 2 in, 2 out]
      }
      event Value Change {
        w7544 = T8."Disabled" ("無効")
        # "⑤"
        # "※複製時\n①このボタンで操作する以外の\n測定旧値\n測定新値\nを複製して作る\n②ある分だけの\n測定旧値\nを複製して作る\n③ある分だけの\n測定旧値\nを複製して作る\n④はそのまま\n⑤測定新値の\nボタンが複製されているか確認\n⑥Ⅰ.初期設定の\n測定新値_リセットの初期化\nを必ず作る事\n⑦キュー"
        n5108 = event-data() -> ("NewVal"=w7553:T7)  [unwired: 1 in, 2 out]
        "測定新値 4" <- w7553
        n5109 = local read "書込周期/ms"() -> (w7543:dbl)
        n5110 = Wait (ms)(milliseconds to wait=w7543) -> ()  [unwired: 1 out]
        n5111 = flat-sequence {
          tunnel: w7553 -> [w7573]
          tunnel: w7554 -> [w7574]
          tunnel: w7556 -> [w7575]
          tunnel: [w7575] -> w7549
          tunnel: [w7574] -> w7548
          tunnel: [w7573] -> w7547
          tunnel: [w7572] -> w7546
          tunnel: [w7625] -> w7552
          tunnel: [w7624] -> w7551
          tunnel: [w7623] -> w7550
          tunnel: w7546 -> [w7622]
          tunnel: w7547 -> [w7623]
          tunnel: w7548 -> [w7624]
          tunnel: w7549 -> [w7625]
          tunnel: [w7646] -> w7557
          tunnel: [w7644] -> w7555
          tunnel: w7552 -> [w7645]
          tunnel: w7551 -> [w7643]
          tunnel: w7550 -> [w7642]
          frame #0 {
            w7572 = 32
            # "測定旧値・新値～32までTrueだったらMAX/MINグローバルリセット"
            # "①"
            n5112 = for {
              N: w7572 -> [_]
              i -> [w7576]
              n5113 = case shown="11" w7576 {
                frame 0, Default {
                  n5114 = local read "測定新値\nリセット用 1"() -> (w7577:bool)
                  n5115 = local read "測定旧値 1"() -> (w7578:bool)
                  n5116 = case shown="TRUE" w7577 {
                    frame False {
                    }
                    frame True {
                      n5117 = property on="MAX/MINグローバルリセット用" class="Arr (指定)"() -> ("Value"=w7579:string[][])  [unwired: 2 in, 2 out]
                      n5118 = global write "測定値MAXMIN_G.vi" "測定値MAX/MINグローバル"(w7579) -> ()
                    }
                  }
                  n5119 = case shown="TRUE" w7578 {
                    frame False {
                    }
                    frame True {
                      n5120 = property on="MAX/MINグローバルリセット用" class="Arr (指定)"() -> ("Value"=w7580:string[][])  [unwired: 2 in, 2 out]
                      n5121 = global write "測定値MAXMIN_G.vi" "測定値MAX/MINグローバル"(w7580) -> ()
                    }
                  }
                }
                frame 1 {
                  n5122 = local read "測定新値\nリセット用 2"() -> (w7581:bool)
                  n5123 = local read "測定旧値 2"() -> (w7582:bool)
                  n5124 = case shown="TRUE" w7581 {
                    frame False {
                    }
                    frame True {
                      n5125 = property on="MAX/MINグローバルリセット用" class="Arr (指定)"() -> ("Value"=w7583:string[][])  [unwired: 2 in, 2 out]
                      n5126 = global write "測定値MAXMIN_G.vi" "測定値MAX/MINグローバル"(w7583) -> ()
                    }
                  }
                  n5127 = case shown="TRUE" w7582 {
                    frame False {
                    }
                    frame True {
                      n5128 = property on="MAX/MINグローバルリセット用" class="Arr (指定)"() -> ("Value"=w7584:string[][])  [unwired: 2 in, 2 out]
                      n5129 = global write "測定値MAXMIN_G.vi" "測定値MAX/MINグローバル"(w7584) -> ()
                    }
                  }
                }
                frame 2 {
                  n5130 = local read "測定新値\nリセット用 3"() -> (w7585:bool)
                  n5131 = local read "測定旧値 3"() -> (w7586:bool)
                  n5132 = case shown="TRUE" w7585 {
                    frame False {
                    }
                    frame True {
                      n5133 = property on="MAX/MINグローバルリセット用" class="Arr (指定)"() -> ("Value"=w7587:string[][])  [unwired: 2 in, 2 out]
                      n5134 = global write "測定値MAXMIN_G.vi" "測定値MAX/MINグローバル"(w7587) -> ()
                    }
                  }
                  n5135 = case shown="TRUE" w7586 {
                    frame False {
                    }
                    frame True {
                      n5136 = property on="MAX/MINグローバルリセット用" class="Arr (指定)"() -> ("Value"=w7588:string[][])  [unwired: 2 in, 2 out]
                      n5137 = global write "測定値MAXMIN_G.vi" "測定値MAX/MINグローバル"(w7588) -> ()
                    }
                  }
                }
                frame 4 {
                  n5138 = local read "測定新値\nリセット用 5"() -> (w7589:bool)
                  n5139 = local read "測定旧値 5"() -> (w7590:bool)
                  n5140 = case shown="TRUE" w7589 {
                    frame False {
                    }
                    frame True {
                      n5141 = property on="MAX/MINグローバルリセット用" class="Arr (指定)"() -> ("Value"=w7591:string[][])  [unwired: 2 in, 2 out]
                      n5142 = global write "測定値MAXMIN_G.vi" "測定値MAX/MINグローバル"(w7591) -> ()
                    }
                  }
                  n5143 = case shown="TRUE" w7590 {
                    frame False {
                    }
                    frame True {
                      n5144 = property on="MAX/MINグローバルリセット用" class="Arr (指定)"() -> ("Value"=w7592:string[][])  [unwired: 2 in, 2 out]
                      n5145 = global write "測定値MAXMIN_G.vi" "測定値MAX/MINグローバル"(w7592) -> ()
                    }
                  }
                }
                frame 5 {
                  n5146 = local read "測定新値\nリセット用 6"() -> (w7593:bool)
                  n5147 = local read "測定旧値 6"() -> (w7594:bool)
                  n5148 = case shown="TRUE" w7593 {
                    frame False {
                    }
                    frame True {
                      n5149 = property on="MAX/MINグローバルリセット用" class="Arr (指定)"() -> ("Value"=w7595:string[][])  [unwired: 2 in, 2 out]
                      n5150 = global write "測定値MAXMIN_G.vi" "測定値MAX/MINグローバル"(w7595) -> ()
                    }
                  }
                  n5151 = case shown="TRUE" w7594 {
                    frame False {
                    }
                    frame True {
                      n5152 = property on="MAX/MINグローバルリセット用" class="Arr (指定)"() -> ("Value"=w7596:string[][])  [unwired: 2 in, 2 out]
                      n5153 = global write "測定値MAXMIN_G.vi" "測定値MAX/MINグローバル"(w7596) -> ()
                    }
                  }
                }
                frame 6 {
                  n5154 = local read "測定新値\nリセット用 7"() -> (w7597:bool)
                  n5155 = local read "測定旧値 7"() -> (w7598:bool)
                  n5156 = case shown="TRUE" w7597 {
                    frame False {
                    }
                    frame True {
                      n5157 = property on="MAX/MINグローバルリセット用" class="Arr (指定)"() -> ("Value"=w7599:string[][])  [unwired: 2 in, 2 out]
                      n5158 = global write "測定値MAXMIN_G.vi" "測定値MAX/MINグローバル"(w7599) -> ()
                    }
                  }
                  n5159 = case shown="TRUE" w7598 {
                    frame False {
                    }
                    frame True {
                      n5160 = property on="MAX/MINグローバルリセット用" class="Arr (指定)"() -> ("Value"=w7600:string[][])  [unwired: 2 in, 2 out]
                      n5161 = global write "測定値MAXMIN_G.vi" "測定値MAX/MINグローバル"(w7600) -> ()
                    }
                  }
                }
                frame 7 {
                  n5162 = local read "測定新値\nリセット用 8"() -> (w7601:bool)
                  n5163 = local read "測定旧値 8"() -> (w7602:bool)
                  n5164 = case shown="TRUE" w7601 {
                    frame False {
                    }
                    frame True {
                      n5165 = property on="MAX/MINグローバルリセット用" class="Arr (指定)"() -> ("Value"=w7603:string[][])  [unwired: 2 in, 2 out]
                      n5166 = global write "測定値MAXMIN_G.vi" "測定値MAX/MINグローバル"(w7603) -> ()
                    }
                  }
                  n5167 = case shown="TRUE" w7602 {
                    frame False {
                    }
                    frame True {
                      n5168 = property on="MAX/MINグローバルリセット用" class="Arr (指定)"() -> ("Value"=w7604:string[][])  [unwired: 2 in, 2 out]
                      n5169 = global write "測定値MAXMIN_G.vi" "測定値MAX/MINグローバル"(w7604) -> ()
                    }
                  }
                }
                frame 8 {
                  n5170 = local read "測定新値\nリセット用 9"() -> (w7605:bool)
                  n5171 = local read "測定旧値 9"() -> (w7606:bool)
                  n5172 = case shown="TRUE" w7605 {
                    frame False {
                    }
                    frame True {
                      n5173 = property on="MAX/MINグローバルリセット用" class="Arr (指定)"() -> ("Value"=w7607:string[][])  [unwired: 2 in, 2 out]
                      n5174 = global write "測定値MAXMIN_G.vi" "測定値MAX/MINグローバル"(w7607) -> ()
                    }
                  }
                  n5175 = case shown="TRUE" w7606 {
                    frame False {
                    }
                    frame True {
                      n5176 = property on="MAX/MINグローバルリセット用" class="Arr (指定)"() -> ("Value"=w7608:string[][])  [unwired: 2 in, 2 out]
                      n5177 = global write "測定値MAXMIN_G.vi" "測定値MAX/MINグローバル"(w7608) -> ()
                    }
                  }
                }
                frame 9 {
                  n5178 = local read "測定新値\nリセット用 10"() -> (w7609:bool)
                  n5179 = local read "測定旧値 10"() -> (w7610:bool)
                  n5180 = case shown="TRUE" w7609 {
                    frame False {
                    }
                    frame True {
                      n5181 = property on="MAX/MINグローバルリセット用" class="Arr (指定)"() -> ("Value"=w7611:string[][])  [unwired: 2 in, 2 out]
                      n5182 = global write "測定値MAXMIN_G.vi" "測定値MAX/MINグローバル"(w7611) -> ()
                    }
                  }
                  n5183 = case shown="TRUE" w7610 {
                    frame False {
                    }
                    frame True {
                      n5184 = property on="MAX/MINグローバルリセット用" class="Arr (指定)"() -> ("Value"=w7612:string[][])  [unwired: 2 in, 2 out]
